vi "Main.vi"() -> ()   [LabVIEW 2014, in "Array Example.lvlib"]
uses:
  Array Example.lvlib
  OOPanel/ArrayManager/ArrayManager.lvclass
  Element B/Element B.lvclass
  Element Base/Element Base.lvclass
  Element A/Element A.lvclass
panel:
  out "Values":string[](array[string])
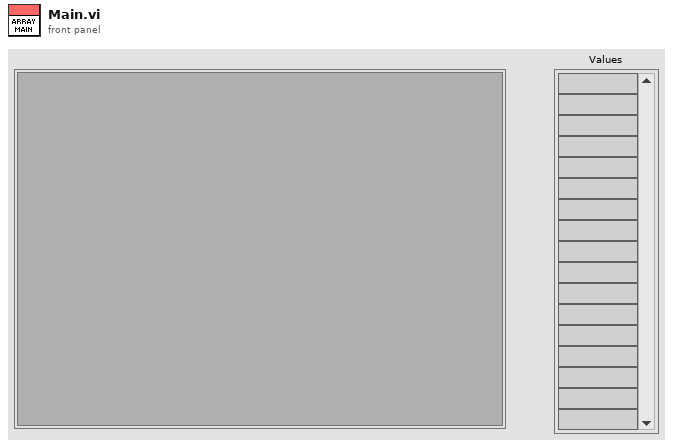
[diagram p1: front panel]
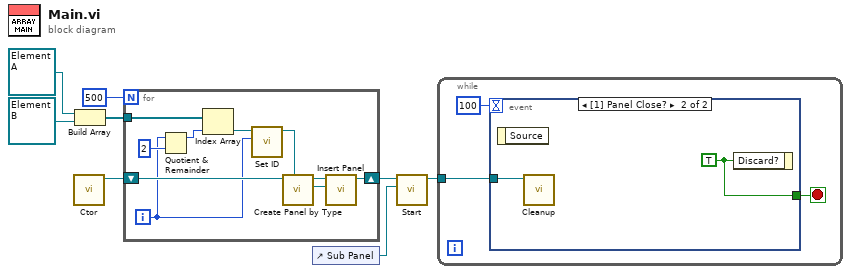
[diagram p0: block diagram]
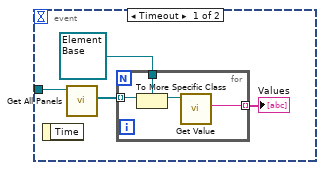
[diagram p2: hidden frame]
diagram:
  n1 = call "Ctor.vi"() -> ("PanelArray"=w8:refnum<class "ArrayManager.lvclass">)  [unwired: 10 in, 1 out]
  n2 = Build Array(refnum<class "Element A.lvclass"> refnum ("Array Example.lvlib:Element A.lvclass"), refnum<class "Element B.lvclass"> refnum ("Array Example.lvlib:Element B.lvclass")) -> (w6:refnum<class "Element Base.lvclass">[])
  n3 = for {
    N: 500 -> [_]
    tunnel: w6 -> [w17]
    shift-right: [w12] -> w4
    shift-left: w8 -> [w15]
    i -> [w13]
    n4 = Quotient & Remainder(x=w13, y=2) -> (x-y*floor(x/y)=w16:i32)  [unwired: 1 out]
    n5 = Index Array(array=w17, index=w16) -> (element=w11:refnum<class "Element Base.lvclass">)
    n6 = call "Set ID.vi"("ID"=w13, "Element Base in"=w11) -> ("Element Base out"=w10:refnum<class "Element Base.lvclass">)  [unwired: 8 in, 1 out]
    n7 = call "Create Panel by Type.vi"("Panel Type"=w10, "PanelArray in"=w15) -> ("Panel"=w9:refnum<class "Element Base.lvclass">, "PanelArray out"=w14:refnum<class "ArrayManager.lvclass">)  [unwired: 7 in, 1 out]
    n8 = call "Insert Panel.vi"("Panel/Type"=w9, "PanelArray in"=w14) -> ("PanelArray out"=w12:refnum<class "ArrayManager.lvclass">)  [unwired: 7 in, 2 out]
  }
  n9 = control-ref of="Sub Panel"() -> (w3:refnum<vi>)
  n10 = call "Start.vi"("Container"=w3, "ArrayManager in"=w4) -> ("ArrayManager out"=w2:refnum<class "ArrayManager.lvclass">)  [unwired: 8 in, 1 out]
  n11 = while {
    tunnel: w2 -> [w20]
    stop <- w19 stop-if-true
    n12 = event shown="[1] Panel Close?" {
      selector: _ -> [_ _]
      dyn-events: _ -> [_ _]
      timeout: 100 -> [_ _]
      tunnel: w20 -> [w25 w30]
      tunnel: [_ w31] -> w19
      event Timeout {
        n13 = event-data() -> ()  [unwired: 1 in, 1 out]
        n14 = call "Get All Panels.vi"("PanelArray in"=w25) -> ("Panels"=w24:refnum<class "ArrayPanel.lvclass">[])  [unwired: 8 in, 2 out]
        n15 = for {
          tunnel: w24 -> [w29] mode=indexing
          tunnel: refnum<class "Element Base.lvclass"> refnum ("Array Example.lvlib:Element Base.lvclass") -> [w28]
          tunnel: [w26] -> w22 mode=indexing
          n16 = To More Specific Class(target class=w28, reference=w29) -> (specific class reference=w27:refnum<class "Element Base.lvclass">)  [unwired: 1 in, 1 out]
          n17 = call-dynamic "Get Value.vi"("Element Base in"=w27) -> ("Value"=w26:string)  [unwired: 8 in, 2 out]
        }
        "Values" <- w22
      }
      event Panel Close? {
        w31 = TRUE ("Discard?")
        n18 = event-data() -> ()  [unwired: 1 in, 1 out]
        n19 = call "Cleanup.vi"("PanelArray in"=w30) -> ()  [unwired: 10 in, 1 out]
        n20 = event-data("Discard?"=w31) -> ()  [unwired: 1 in, 1 out]
      }
    }
  }
